vi "MachineStatusGV.vi"() -> ()   [LabVIEW 2017]
panel:
  out "MachineOn?":bool
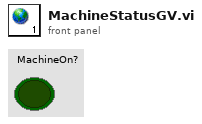
[diagram p1: front panel]
diagram:
